vi "ifr2025 Operating Time  .vi"(8 "error in (no error)":errorcluster {"code" format="%.0x"}, 11 "instrument handle":refnum<visa-resource-name>) -> (0 "error out":errorcluster {"code" format="%.0x"}, 2 "Operating Hours":dbl, 3 "instrument handle out":refnum<visa-resource-name>)   [LabVIEW 2009]
doc: "This VI reads the total number of operating hours on the instrument, e.g. 1453.00"
uses:
  Ifr2025_32.dll
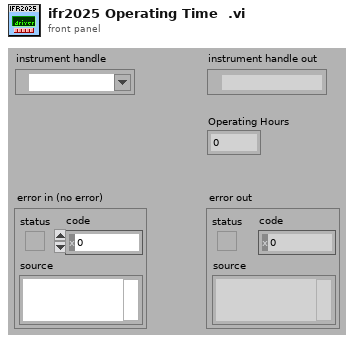
[diagram p1: front panel]
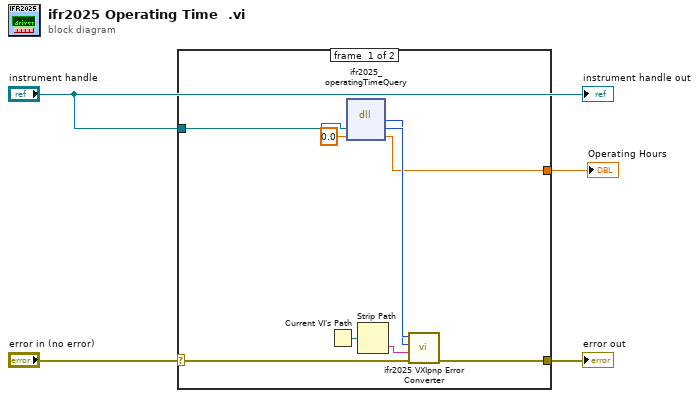
[diagram p0: block diagram]
diagram:
  n1 = case shown="No Error" "error in (no error)" {
    selector: "error in (no error)" -> [w8 w14]
    tunnel: [w7 w14] -> w4
    tunnel: "instrument handle" -> [w12 _]
    tunnel: [w5 _] -> w1
    frame #0 {
      n2 = Current VI's Path() -> (path=w13:path)
      n3 = dll-call lib="P:/inst/Marconi 2024 Signal Generator/source/labview/ifr2025/ifr2025/ifr2025_*.*" fn="ifr2025_operatingTimeQuery"("vi"=w12, "Operating Hours"=0.0) -> (w10:i32, "vi"=w11:u32, "Operating Hours"=w5:dbl)  [unwired: 3 in, 2 out]
      n4 = Strip Path(path=w13) -> (name=w9:string)  [unwired: 1 out]
      n5 = call "ifr2025 VXIpnp Error Converter.vi"("error in (no error)"=w8, "name of VI (\"\")"=w9, "CVI error code (0)"=w10, "instrument handle"=w11) -> ("error out"=w7:errorcluster)  [unwired: 7 out]
    }
    frame #1 {
    }
  }
  "error out" <- w4
  "Operating Hours" <- w1
  "instrument handle out" <- "instrument handle"
